vi "test CRUD stage.vi"() -> ()   [LabVIEW 2019]
uses:
  Controls/JSON - Stage.ctl
  <vilib>/httpClient/POSTBuffer.vi
  <vilib>/httpClient/LabVIEWHTTPClient.lvlib
panel:
  out "Table C 2":string[][](table)=[["1", "1", "1", "1"], ["2", "2", "2", "2"], ["3", "3", "3", "3"], ["4", "4", "4", "4"]]
  in  "Table C":string[][](table)=[["1", "1", "1", "1"], ["2", "2", "2", "2"], ["3", "3", "3", "3"], ["4", "4", "4", "4"]]
  out "body":string
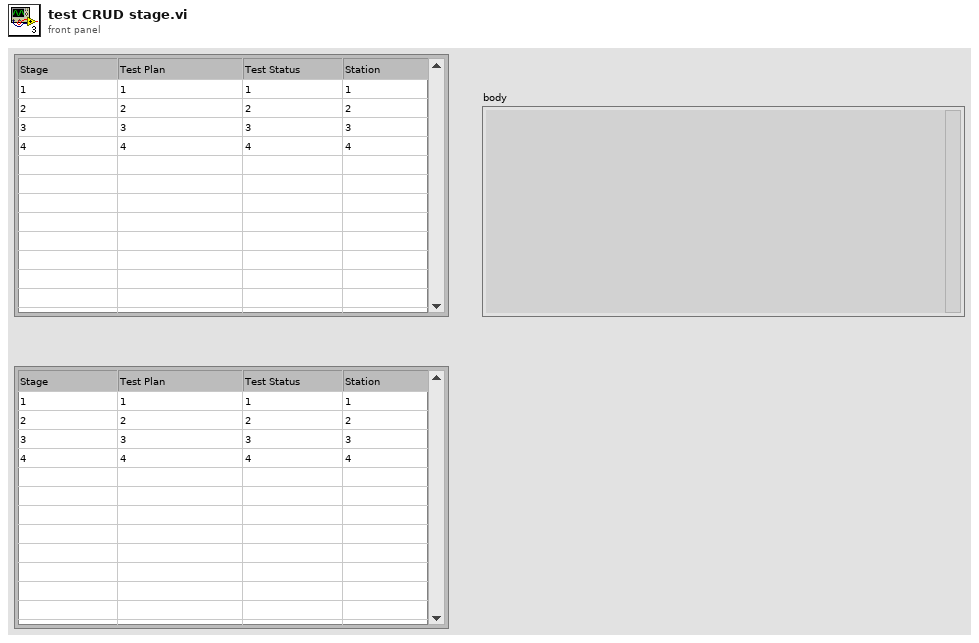
[diagram p1: front panel]
types:
  T1 = cluster{"filename":string, "stage":string, "action":string, "testplan":string, "station":string, "status":string}
  T2 = typedef "JSON - Stage.ctl" = cluster{"status":string, "data":cluster{"id":string, "created_date":string, "filename":string, "stage":string, "testplan":string, "station":string, "status":string, "delete":string}[]}
  T3 = typedef "LabVIEWHTTPClient.lvlib/ClientHandle.ctl" = refnum<k1>
  T4 = cluster{"id":string, "created_date":string, "filename":string, "stage":string, "testplan":string, "station":string, "status":string, "delete":string}[]
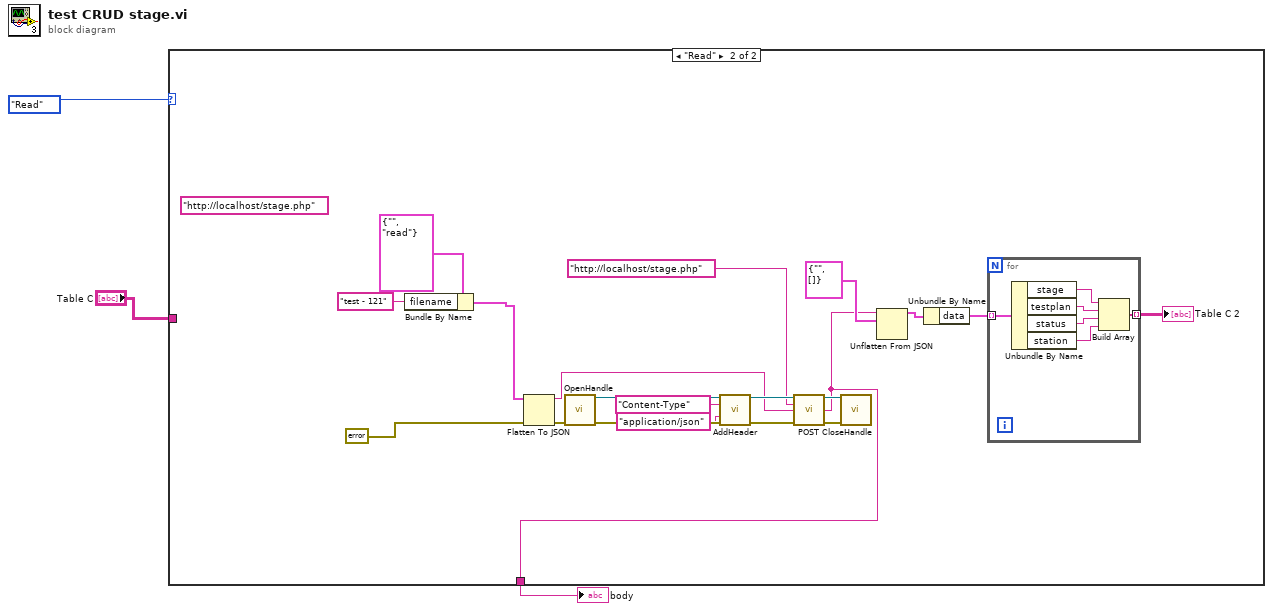
[diagram p0: block diagram]
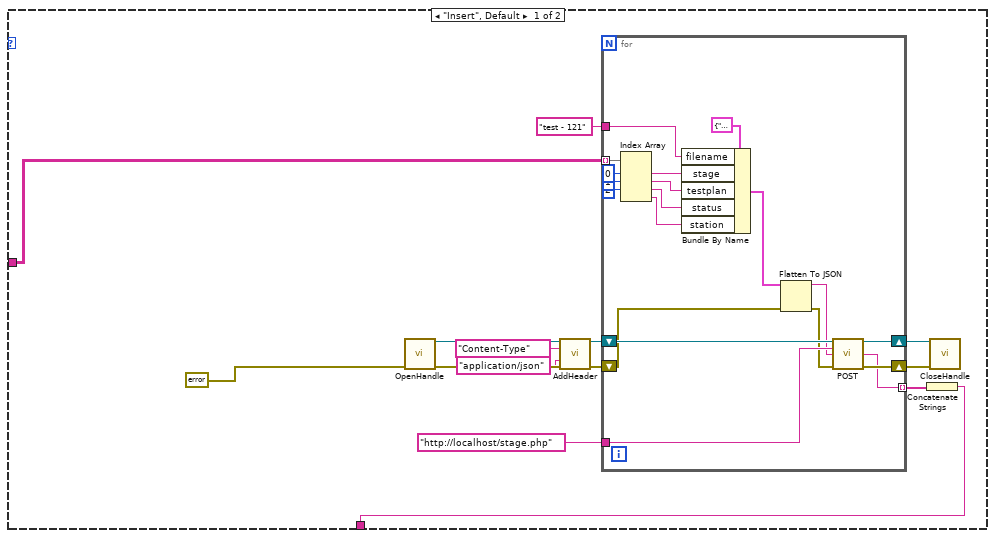
[diagram p2: hidden frame]
diagram:
  n1 = case shown="\"Read\"" enum16{"Insert", "Read", "Delete", "Update"}."Read" {
    tunnel: [w5 w40] -> w2
    tunnel: "Table C" -> [w7 _]
    frame "Insert", Default {
      n2 = call <vilib>:"OpenHandle.vi"("error in (no error)"=errorcluster {"status"=FALSE, "code"=0, "source"=""} ("error IO")) -> ("client handle out"=w16:T3, "error out"=w17:errorcluster)  [unwired: 13 in]
      n3 = call <vilib>:"AddHeader.vi"("client handle"=w16, "header"="Content-Type", "value"="application/json", "error in (no error)"=w17) -> ("client handle out"=w10:T3, "error out"=w13:errorcluster)  [unwired: 10 in]
      n4 = for {
        tunnel: "http://localhost/stage.php" ("url") -> [w33]
        tunnel: "test - 121" ("Filename") -> [w29]
        shift-right: [w34] -> w11
        shift-left: w10 -> [w35]
        shift-right: [w36] -> w12
        shift-left: w13 -> [w30]
        tunnel: w7 -> [w28] mode=indexing
        tunnel: [w19] -> w6 mode=indexing
        n5 = Index Array(array=w28, index #1=0 ("index"), index #2=1 ("index"), index #3=2 ("index")) -> (element #1=w27:string, element #2=w26:string, element #3=w22:string, element #4=w18:string)  [unwired: 1 in]
        n6 = Bundle By Name(cluster=T1 {"filename"="", "stage"="", "action"="insert", "testplan"="", "station"="", "status"=""}, "filename"=w29, "stage"=w27, "testplan"=w26, "status"=w22, "station"=w18) -> (w31:T1)
        n7 = Flatten To JSON(anything=w31, error in (no error)=w30) -> (JSON string=w20:string, 11:w21:errorcluster)  [unwired: 1 in]
        n8 = call-poly <vilib>:"POST.vi"("client handle"=w35, "url"=w33, "buffer"=w20, "error in (no error)"=w21) -> ("client handle out"=w34:T3, "body"=w19:string, "error out"=w36:errorcluster)  [unwired: 8 in, 1 out]
      }
      n9 = Concatenate Strings(w6) -> (w5:string)
      n10 = call <vilib>:"CloseHandle.vi"("client handle"=w11, "error in (no error)"=w12) -> ()  [unwired: 13 in, 1 out]
    }
    frame "Read" {
      (unwired) "http://localhost/stage.php" ("url")
      n11 = Bundle By Name(cluster=cluster{"filename":string, "action":string} {"filename"="", "action"="read"}, "filename"="test - 121") -> (w43:cluster{"filename":string, "action":string})
      n12 = Flatten To JSON(anything=w43, error in (no error)=errorcluster {"status"=FALSE, "code"=0, "source"=""} ("error IO")) -> (JSON string=w45:string, 11:w46:errorcluster)  [unwired: 1 in]
      n13 = call <vilib>:"OpenHandle.vi"("error in (no error)"=w46) -> ("client handle out"=w53:T3, "error out"=w55:errorcluster)  [unwired: 13 in]
      n14 = call <vilib>:"AddHeader.vi"("client handle"=w53, "header"="Content-Type", "value"="application/json", "error in (no error)"=w55) -> ("client handle out"=w52:T3, "error out"=w54:errorcluster)  [unwired: 10 in]
      n15 = call-poly <vilib>:"POST.vi"("client handle"=w52, "url"="http://localhost/stage.php", "buffer"=w45, "error in (no error)"=w54) -> ("client handle out"=w47:T3, "body"=w40:string, "error out"=w48:errorcluster)  [unwired: 8 in, 1 out]
      n16 = call <vilib>:"CloseHandle.vi"("client handle"=w47, "error in (no error)"=w48) -> ()  [unwired: 13 in, 1 out]
      n17 = Unflatten From JSON(JSON string=w40, type and defaults=T2 {"status"="", "data"=[]}) -> (value=w39:T2)  [unwired: 5 in, 1 out]
      n18 = Unbundle By Name(w39) -> ("data"=w38:T4)
      n19 = for {
        tunnel: w38 -> [w62] mode=indexing
        tunnel: [w57] -> w37 mode=indexing
        n20 = Unbundle By Name(w62) -> ("stage"=w61:string, "testplan"=w60:string, "status"=w59:string, "station"=w58:string)
        n21 = Build Array(w61, w60, w59, w58) -> (w57:string[])
      }
      "Table C 2" <- w37
    }
  }
  "body" <- w2
